vi "WriteL.vi"(0 "val":u32, 1 "offset":u32) -> ()   [LabVIEW 2015]
uses:
  lwlscdll.dll
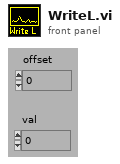
[diagram p1: front panel]
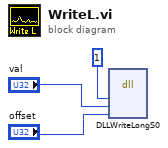
[diagram p0: block diagram]
diagram:
  n1 = dll-call lib="G:/SD/IR-det/lv/2cam/board.vis/lwlscdll.dll" fn="DLLWriteLongS0"("drv"=u32 1, "DataByte"="val", "PortOff"="offset") -> ()  [unwired: 7 in, 2 out]
